vi "Shutter.vi"(1 "Shutter":enum16{"OPEN", "CLOSE"}(ring)) -> (0 "Error":bool)   [LabVIEW 2014]
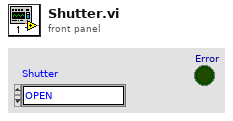
[diagram p1: front panel]
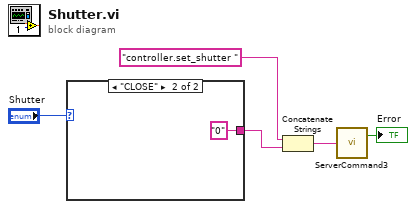
[diagram p0: block diagram]
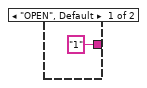
[diagram p2: hidden frame]
diagram:
  n1 = case shown="\"CLOSE\"" "Shutter" {
    tunnel: ["1" "0"] -> w1
    frame "OPEN", Default {
    }
    frame "CLOSE" {
    }
  }
  n2 = Concatenate Strings("controller.set_shutter ", w1) -> (w2:string)
  n3 = call "ServerCommand3.vi"("Command"=w2) -> ("Error"=→"Error":bool)  [unwired: 1 out]
